vi "INTELLIFAUCET Temp-Flow.vi"(8 "Error In":errorcluster, 10 "TEMP,FLOW":T1, 11 "VISA session":refnum<visa-resource-name>="MW100") -> (0 "Error Out":errorcluster, 3 "dup VISA session":refnum<visa-resource-name>)   [LabVIEW 2016]
uses:
  Type Definitions/INTELLIFAUCT Temp Flow.ctl
  MW100/Type Definitions/HEWH MW100 Channel Numbers.ctl
  Type Definitions/HEWH Normally Open Valve Control.ctl
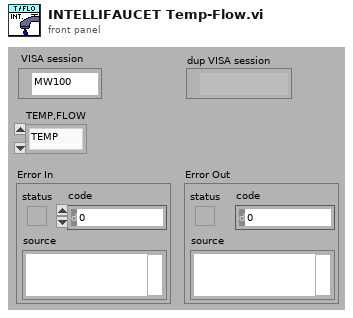
[diagram p1: front panel]
types:
  T1 = typedef "INTELLIFAUCT Temp Flow.ctl" = enum8{"TEMP", "FLOW"}
  T2 = typedef "HEWH MW100 Channel Numbers.ctl" = string
  T3 = typedef "HEWH Normally Open Valve Control.ctl" = string
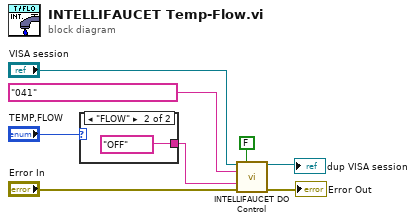
[diagram p0: block diagram]
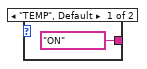
[diagram p2: hidden frame]
diagram:
  n1 = case shown="\"FLOW\"" "TEMP,FLOW" {
    tunnel: [T3 "ON" ("Normally Open Valve") T3 "OFF" ("Normally Open Valve")] -> w1
    frame "TEMP", Default {
    }
    frame "FLOW" {
    }
  }
  n2 = call "INTELLIFAUCET DO Control.vi"("VISA session"="VISA session", "Normally Closed Valve?"=FALSE, "HEWH MW100 Channel Numbers"=T2 "041", "Normally Open Valve"=w1, "Error In"="Error In") -> ("dup VISA session"=→"dup VISA session":refnum<visa-resource-name>, "error out"=→"Error Out":errorcluster)  [unwired: 7 in, 2 out]
